vi "_FPGA Syringe Control.vi"(4 "Timeout (2s)":u32=2000, 5 "error in (no error)":errorcluster, 6 "Input Value":sgl, 7 "Pump Command":T1=enum."status") -> (0 "error out":errorcluster, 2 "Reply":string)   [LabVIEW 2012]
uses:
  Type/_Syringe Pump Command.ctl
  Type/_RT Serial Command.ctl
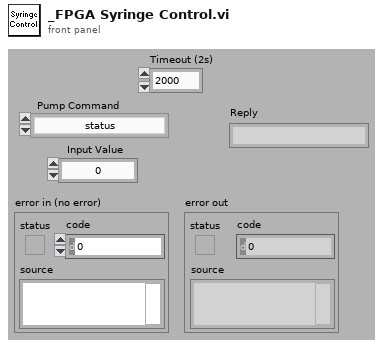
[diagram p1: front panel]
types:
  T1 = typedef "_Syringe Pump Command.ctl" = enum16{"start", "stop", "pause", "restart", "help", "set units", "set diameter", "set rate", "set time", "set volume", "set delay", "save setting", "read limit parameter", "view parameter", "status"}
  T2 = typedef "_RT Serial Command.ctl" = cluster{"Port Type":u16, "baud rate (9600)":u32, "data bits (8)":u16, "stop bits (1)":u16, "parity (0:none)":u16, "DoRead":bool, "Command":string}
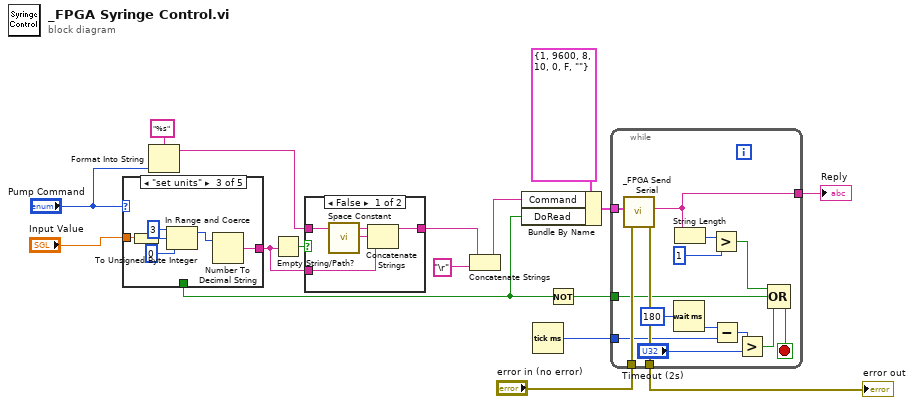
[diagram p0: block diagram]
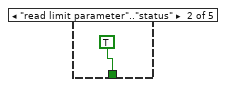
[diagram p4: hidden frame]
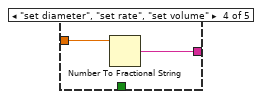
[diagram p5: hidden frame]
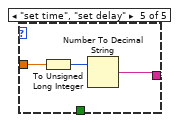
[diagram p6: hidden frame]
diagram:
  n1 = case shown="\"set units\"" "Pump Command" {
    tunnel: "Input Value" -> [_ _ w24 w26 w28]
    tunnel: [_ _ w22 w25 w27] -> w6
    tunnel: [_ TRUE _ _ _] -> w4
    frame Default {
    }
    frame "read limit parameter".."status" {
    }
    frame "set units" {
      n2 = To Unsigned Byte Integer(number=w24) -> (unsigned 8bit integer=w23:u8)
      n3 = In Range and Coerce(upper limit=u8 3, x=w23, lower limit=u8 0) -> (coerced(x)=w21:u8)  [unwired: 1 out]
      n4 = Number To Decimal String(number=w21) -> (decimal integer string=w22:string)  [unwired: 1 out]
    }
    frame "set diameter", "set rate", "set volume" {
      n5 = Number To Fractional String(number=w26) -> (F-format string=w25:string)  [unwired: 3 out]
    }
    frame "set time", "set delay" {
      n6 = To Unsigned Long Integer(number=w28) -> (unsigned 32bit integer=w29:u32)
      n7 = Number To Decimal String(number=w29) -> (decimal integer string=w27:string)  [unwired: 1 out]
    }
  }
  n8 = Format Into String(format string="%s", "Pump Command") -> (resulting string=w7:string)  [unwired: 2 in, 1 out]
  n9 = Empty String/Path?(string/path=w6) -> (empty?=w9:bool)
  n10 = case shown="False" w9 {
    tunnel: w6 -> [w31 _]
    tunnel: w7 -> [w33 w34]
    tunnel: [w30 w34] -> w10
    frame False {
      n11 = call <vilib>:"Space Constant.vi"() -> ("String"=w32:string)
      n12 = Concatenate Strings(w33, w32, w31) -> (w30:string)
    }
    frame True {
    }
  }
  n13 = Concatenate Strings(w10, "\r" ("string")) -> (w5:string)
  n14 = Bundle By Name(cluster=T2 {"Port Type"=1, "baud rate (9600)"=9600, "data bits (8)"=8, "stop bits (1)"=10, "parity (0:none)"=0, "DoRead"=FALSE, "Command"=""}, "Command"=w5, "DoRead"=w4) -> (w16:T2)
  n15 = Tick Count (ms)() -> (millisecond timer value=w2:u32)
  n16 = Not(x=w4) -> (.not. x?=w3:bool)
  n17 = while {
    tunnel: w16 -> [w49]
    tunnel: "error in (no error)" -> [w48]
    tunnel: [w47] -> w14
    tunnel: [w38] -> w1
    tunnel: w3 -> [w43]
    tunnel: w2 -> [w41]
    stop <- w44 stop-if-true
    n18 = call "_FPGA Send Serial.vi"("error in"=w48, "Serial Command"=w49) -> ("error out"=w47:errorcluster, "Reply"=w38:string)  [unwired: 2 in, 2 out]
    n19 = Wait (ms)(milliseconds to wait=u32 180) -> (millisecond timer value=w42:u32)
    n20 = String Length(string=w38) -> (length=w37:i32)
    n21 = Greater?(x=w37, y=1) -> (0:w35:bool)
    n22 = Subtract(x=w42, y=w41) -> (x-y=w40:u32)
    n23 = Greater?(x=w40, y="Timeout (2s)") -> (0:w39:bool)
    n24 = Compound Arithmetic op=OR(w35, w43, w39) -> (w44:bool)
  }
  "error out" <- w14
  "Reply" <- w1
